vi "Inverse Real FFT PtByPt.vi"(2 "initialize":bool, 3 "sample length":i32=100, 5 "x":cdb format="%#.6g") -> (0 "error":i32, 1 "Inverse FFT{X}":dbl[](array[numeric]))   [LabVIEW 2017, in "NI_PtbyPt.lvlib"]
doc: "Computes the inverse discrete Fourier transform (IDFT) of the set of input data points specified by <B>sample length</B>. This VI is similar to the Inverse FFT VI. Wire data to the <B>x</B> input to determine the polymorphic instance to use or manually select the instance."
uses:
  <vilib>/ptbypt/NI_PtbyPt.lvlib
  <vilib>/Analysis/1siggen.llb/Ramp Pattern by Samples.vi
  <vilib>/Analysis/NI_AALBase.lvlib
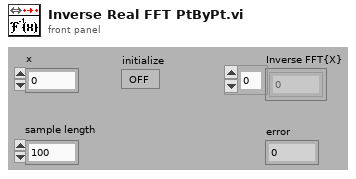
[diagram p1: front panel]
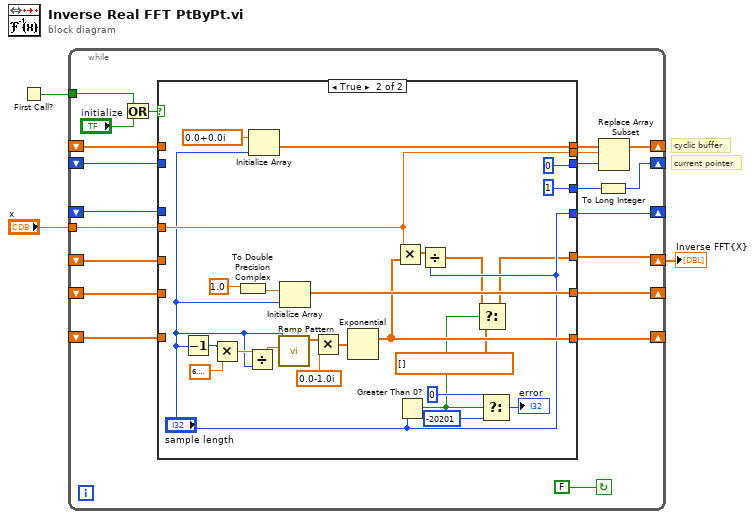
[diagram p0: block diagram]
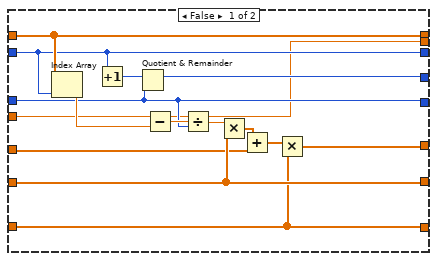
[diagram p2: hidden frame]
diagram:
  # "current pointer"
  # "cyclic buffer"
  n1 = First Call?() -> (First Call?: T/F=w1:bool)
  n2 = while {
    tunnel: w1 -> [w4]
    tunnel: "x" -> [w9]
    shift-left: _ -> [w10]
    shift-right: [w11] -> _
    shift-left: _ -> [w13]
    shift-right: [w12] -> _
    shift-left: _ -> [w19]
    shift-right: [w18] -> _
    shift-left: _ -> [w20]
    shift-right: [w21] -> _
    shift-left: _ -> [w22]
    shift-right: [w24] -> w3
    shift-left: _ -> [w23]
    shift-right: [w16] -> _
    stop <- FALSE continue-if-true
    n3 = Or(x=w4, y="initialize") -> (x .or. y?=w6:bool)
    n4 = case shown="True" w6 {
      tunnel: w10 -> [w26 _]
      tunnel: [w30 w41] -> w24
      tunnel: [w39 w63] -> w17
      tunnel: w23 -> [w39 _]
      tunnel: w22 -> [w33 _]
      tunnel: [w31 w50] -> w21
      tunnel: w20 -> [w31 _]
      tunnel: w19 -> [w36 _]
      tunnel: [w36 w51] -> w18
      tunnel: [w34 0 ("Index")] -> w15
      tunnel: [w27 1 ("Index")] -> w14
      tunnel: w13 -> [w34 _]
      tunnel: [w26 "sample length"] -> w11
      tunnel: w9 -> [w25 w48]
      tunnel: [w25 w48] -> w8
      frame False {
        n5 = Index Array(array=w39, index=w34) -> (element=w38:cdb)
        n6 = Increment(x=w34) -> (x+1=w28:i32)
        n7 = Quotient & Remainder(x=w28, y=w26) -> (x-y*floor(x/y)=w27:i32)  [unwired: 1 out]
        n8 = Subtract(x=w25, y=w38) -> (x-y=w37:cdb)
        n9 = Divide(x=w37, y=w26) -> (x/y=w29:cdb)
        n10 = Multiply(x=w29, y=w36) -> (x*y=w35:cdb[])
        n11 = Add(x=w35, y=w33) -> (x+y=w32:cdb[])
        n12 = Multiply(x=w32, y=w31) -> (x*y=w30:cdb[])
      }
      frame True {
        n13 = Decrement(x="sample length") -> (x-1=w58:i32)
        n14 = Multiply(x=w58, y=6.283185307179586) -> (x*y=w57:dbl)
        n15 = To Double Precision Complex(1:1.0) -> (0:w52:cdb)
        n16 = Divide(x=w57, y="sample length") -> (x/y=w56:dbl)
        n17 = Initialize Array(cdb 0.0+0.0i ("Element Data"), "sample length") -> (w63:cdb[])
        n18 = call-poly <vilib>:"Ramp Pattern.vi"("end"=w56, "samples"="sample length") -> ("Ramp Pattern"=w60:dbl[])  [unwired: 8 in, 1 out]
        n19 = Initialize Array(w52, "sample length") -> (w51:cdb[])
        n20 = Multiply(x=w60, y=cdb 0.0-1.0i) -> (x*y=w53:cdb[])
        n21 = Exponential(1:w53) -> (0:w50:cdb[])
        n22 = Multiply(x=w48, y=w50) -> (x*y=w49:cdb[])
        n23 = Greater Than 0?(x="sample length") -> (x > 0?=w43:bool)
        n24 = Divide(x=w49, y="sample length") -> (x/y=w42:cdb[])
        n25 = Select(t=w42, s=w43, f=cdb[] []) -> (s? t:f=w41:cdb[])
        n26 = Select(t=0, s=w43, f=-20201) -> (s? t:f=→"error":i32)
      }
    }
    n27 = To Long Integer(number=w14) -> (32bit integer=w12:i32)
    n28 = Replace Array Subset(array=w17, new element=w8, index=w15) -> (w16:cdb[])
  }
  "Inverse FFT{X}" <- w3
